vi "FaultClear.vi"(10 "Channel":string, 11 "ChannelFault in":T1) -> (0 "error out":errorcluster, 2 "Channel out":string)   [LabVIEW 2015, in "MiscHelperVIs.lvlib"]
uses:
  MiscHelperVIs.lvlib
  <vilib>/NI Veristand/Execution/ChannelFaultManager/ChannelFaultAPI.ctl
  NationalInstruments.VeriStand.ClientAPI
  <vilib>/NI Veristand/Execution/ChannelFaultManager/NI_VS ChannelFault ExecutionAPI.lvlib
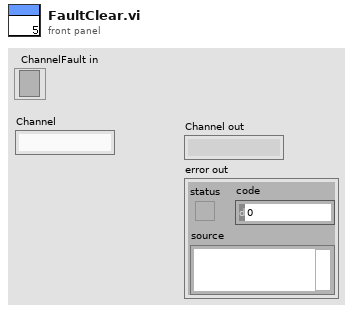
[diagram p1: front panel]
types:
  T1 = typedef "NI_VS ChannelFault ExecutionAPI.lvlib/ChannelFaultAPI.ctl" = refnum<k24>
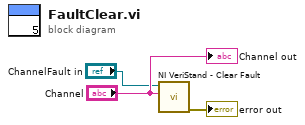
[diagram p0: block diagram]
diagram:
  n1 = call <vilib>:"NI VeriStand - Clear Fault.vi"("Channel"="Channel", "ChannelFault in"="ChannelFault in") -> ("error out"=→"error out":errorcluster)  [unwired: 8 in, 1 out]
  "Channel out" <- "Channel"
